vi "exercise5.vi"() -> ()   [LabVIEW 2020]
uses:
  <vilib>/Utility/file.llb/Read Delimited Spreadsheet (DBL).vi
panel:
  out "Waveform Graph":dbl[](graph)
  out "Wave 2":dbl[](graph)
  out "Wave 1":dbl[](graph)
  out "Phase Shift":dbl
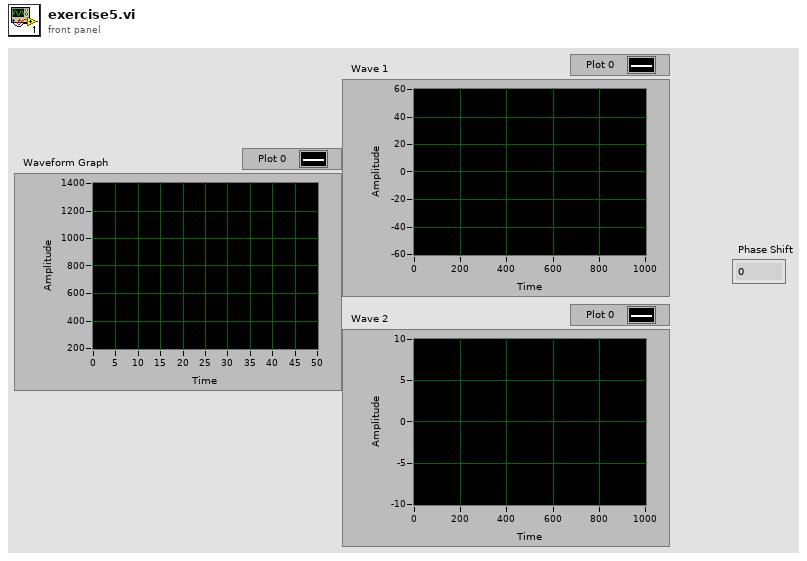
[diagram p1: front panel]
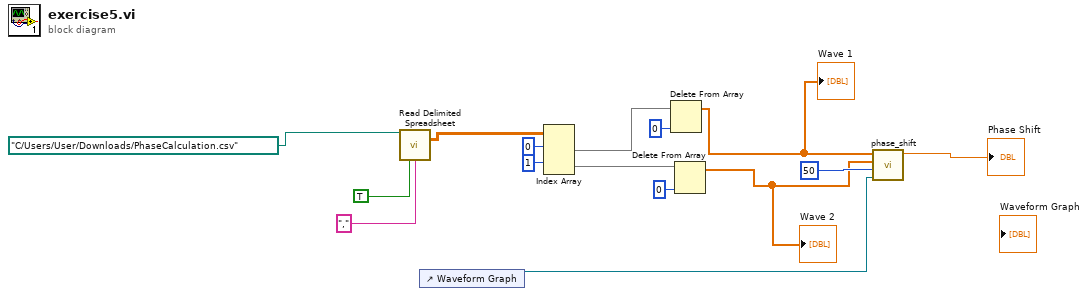
[diagram p0: block diagram]
diagram:
  n1 = call-poly <vilib>:"Read Delimited Spreadsheet.vi"("file path (dialog if empty)"=path "C:/Users/User/Downloads/PhaseCalculation.csv" ("file path (use dialog)"), "transpose? (F)"=TRUE, "delimiter (\\t)"="," ("delimiter (\\t)")) -> ("all rows"=w12:dbl[][])  [unwired: 7 in, 5 out]
  n2 = control-ref of="Waveform Graph"() -> (w8:refnum<vi>)
  n3 = Index Array(array=w12, index (row) #1=0 ("index (row)"), index (row) #2=1 ("index (row)")) -> (element #1=w5:dbl[], element #2=w3:dbl[])  [unwired: 2 in]
  n4 = Delete From Array(array=w5, index=0) -> (array with subset deleted=w4:dbl[])  [unwired: 1 in, 1 out]
  "Wave 1" <- w4
  n5 = Delete From Array(array=w3, index=0) -> (array with subset deleted=w1:dbl[])  [unwired: 1 in, 1 out]
  "Wave 2" <- w1
  n6 = call "phase_shift.vi"("reference"=w8, "Points in Cycle"=50, "Array 2"=w1, "Array 1"=w4) -> ("Phase Shift"=→"Phase Shift":dbl)  [unwired: 7 in]
